vi "BBControl Dialog.vi"(8 "error in (no error)":errorcluster, 11 "BBCont Parameters In":T2 {"BBControl Criteria"."Comparison" items=["<", ">"]}) -> (0 "error out":errorcluster, 1 "Cancelled?":bool=TRUE, 2 "UI Refresh Needed?":bool, 3 "BBCont Parameters Out":T2 {"BBControl Criteria"."Comparison" items=["<", ">"]})   [LabVIEW 2024]
doc: "Dialog for selecting user specified settings."
uses:
  support/Control/BBControl Parameters.ctl
  ef7c00e2-4e74-40b8-8720-694a588d8cdf.vi
  74ebc26f-2795-41b4-bcda-487ba7bbdbc9.vi
  Display/Global 1.vi
  <vilib>/Utility/xml.llb/Write to XML File(string).vi
  <vilib>/Comparison/Equal/Equal Functor/Equal Functor.lvclass
panel:
  in  "Save as Preset":bool
  in  "Load Preset":bool
  in  "BangBang Control":T1(array[cluster]) {"Comparison" items=["<", ">"]}
  in  "Cancel Button":bool
  in  "OK Button":bool
  # "Non visible portion of dialog (needed for connector pane)."
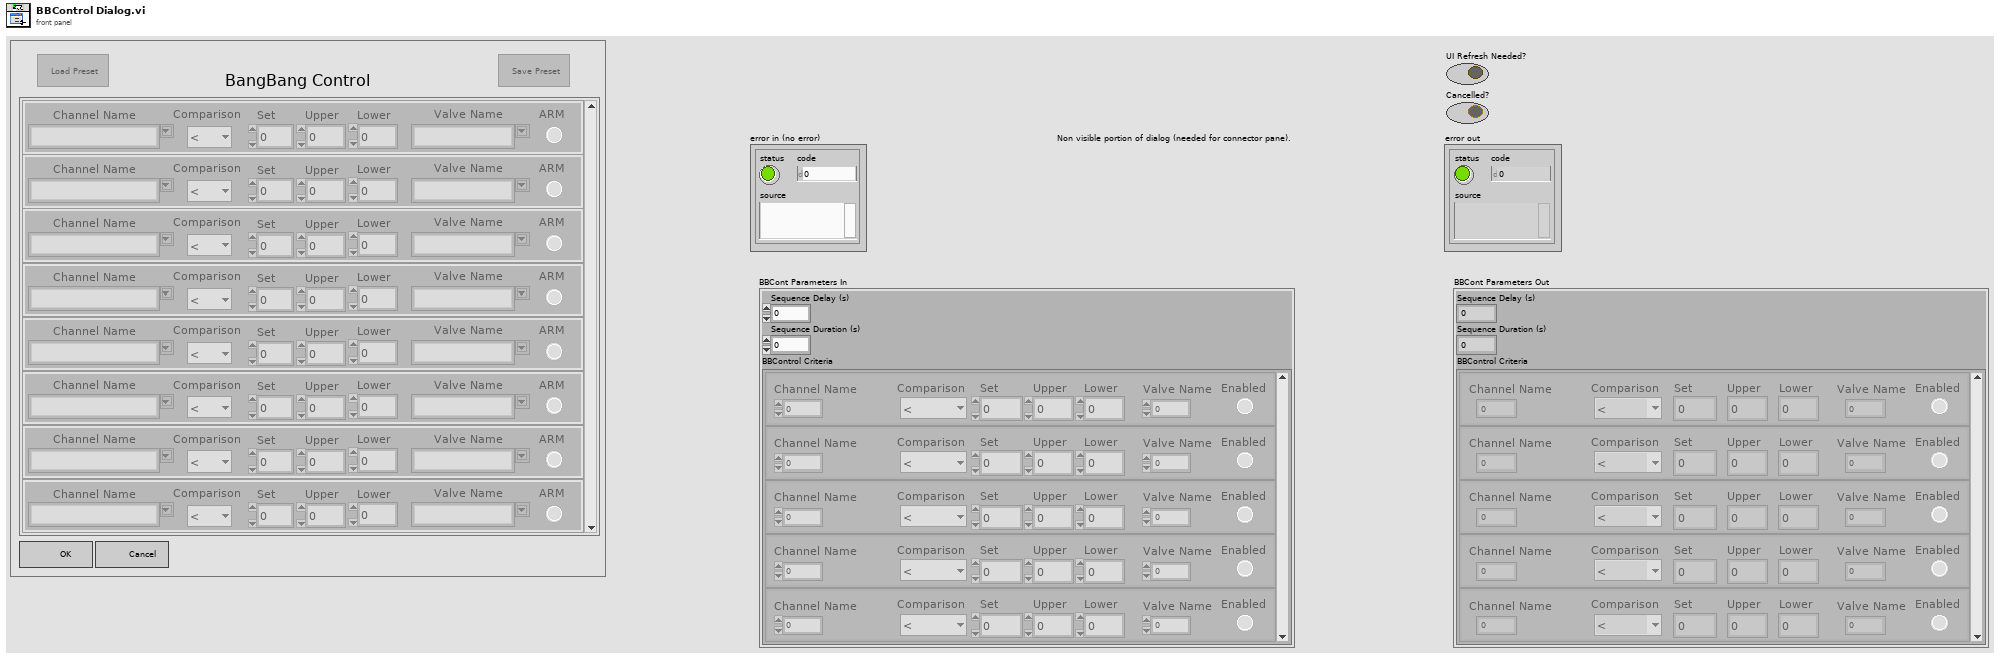
[diagram p1: front panel]
types:
  T1 = cluster{"Channel Name":string, "Comparison\n":u16, "Set":dbl, "ARM":bool, "Valve Name":string, "Upper":dbl, "Lower":dbl}[]
  T2 = typedef "BBControl Parameters.ctl" = cluster{"Sequence Delay (s)":dbl, "Sequence Duration (s)":dbl, "BBControl Criteria":cluster{"Channel Name":i32, "Comparison":u16, "Set":dbl, "Enabled":bool, "Valve Name":i32, "Upper":dbl, "Lower":dbl}[]}
  T3 = cluster{"Channel Name":string, "Comparison":u16, "Set":dbl, "Enabled":bool, "Valve Name":string, "Upper":dbl, "Lower":dbl}
  T4 = cluster{"Channel Name":i32, "Comparison":u16, "Set":dbl, "Enabled":bool, "Valve Name":i32, "Upper":dbl, "Lower":dbl}
  T5 = typedef "Calibration Configuration.ctl" = cluster{"ai Calibration Slope":dbl[], "ai Calibration Offset":dbl[], "ai Sensor Names ":string[], "tc Sensor Names":string[], "di Sensor Names":string[], "do Sensor Names":string[], "bc Sensor Names":string[], "ai Sensor Units":string[], "tc Sensor Units":string[], "bc Sensor Units":string[]}
  T6 = cluster{"Channel Name":i32, "Comparison":u16, "Set":dbl, "Enabled":bool, "Valve Name":i32, "Upper":dbl, "Lower":dbl}[]
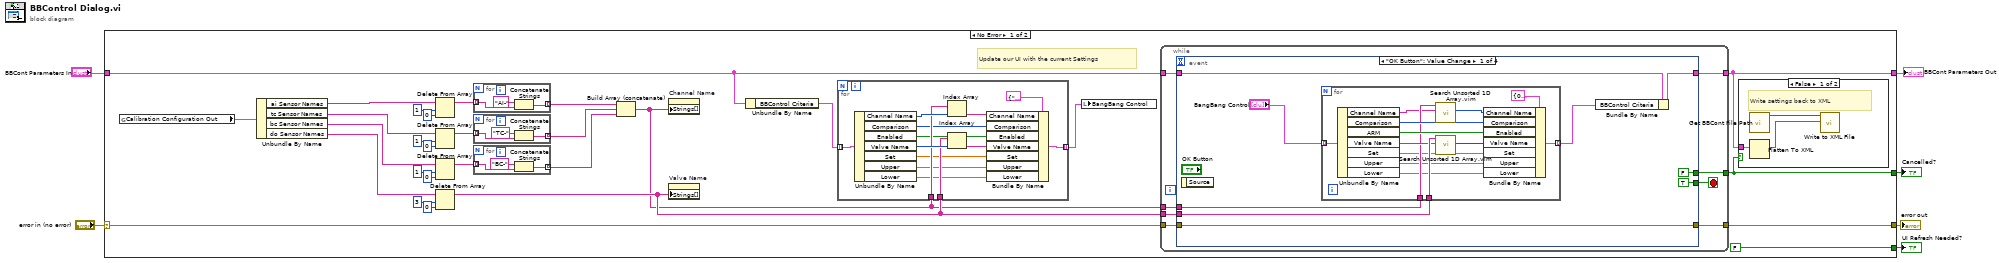
[diagram p0: block diagram]
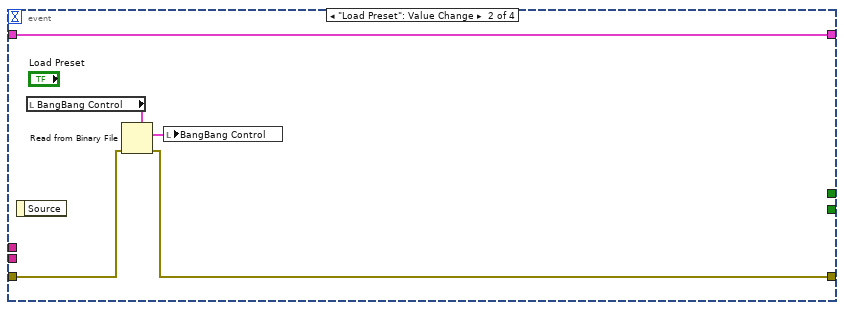
[diagram p3: hidden frame]
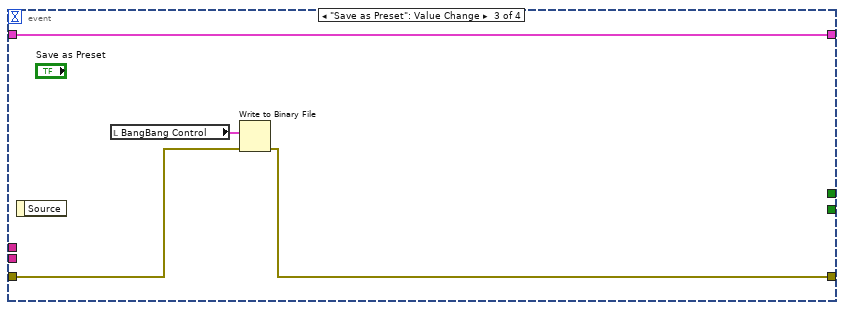
[diagram p4: hidden frame]
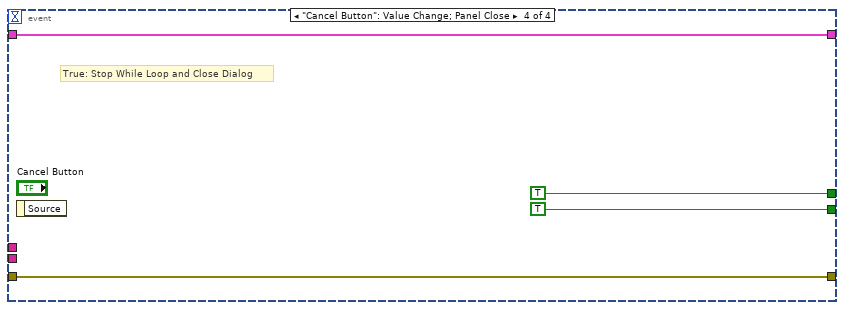
[diagram p5: hidden frame]
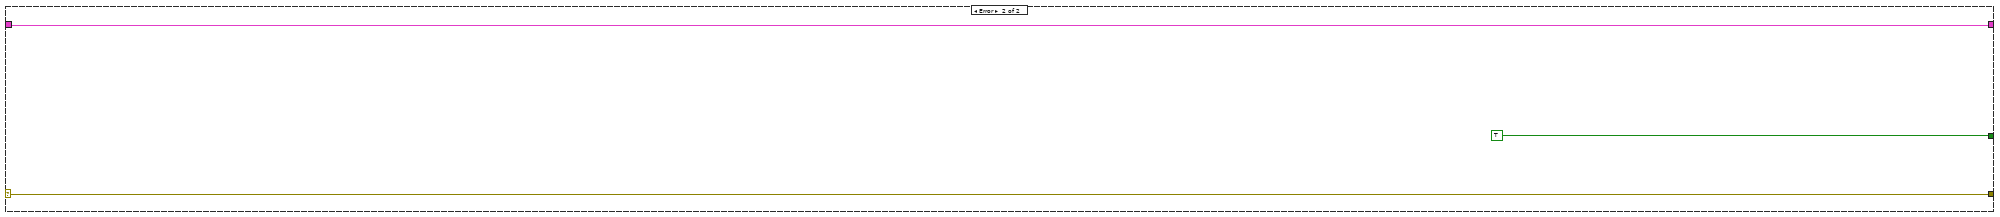
[diagram p6: hidden frame]
diagram:
  n1 = case shown="No Error" "error in (no error)" {
    selector: "error in (no error)" -> [w12 w108]
    tunnel: [w31 w108] -> w6
    tunnel: "BBCont Parameters In" -> [w34 w107]
    tunnel: [w33 w107] -> w1
    tunnel: [FALSE ("UI Refresh Needed?") _] -> w5
    tunnel: [w32 TRUE ("UI Refresh Needed?")] -> w4
    frame No Error {
      # "Update our UI with the current Settings"
      n2 = global read "Global 1.vi" "Calibration Configuration Out"() -> (w15:T5)
      n3 = Unbundle By Name(w15) -> ("ai Sensor Names"=w24:string[], "tc Sensor Names"=w23:string[], "bc Sensor Names"=w22:string[], "do Sensor Names"=w13:string[])
      n4 = Delete From Array(array=w24, length=1, index=0) -> (array with subset deleted=w19:string[])  [unwired: 1 out]
      n5 = Delete From Array(array=w23, length=1, index=0) -> (array with subset deleted=w20:string[])  [unwired: 1 out]
      n6 = Delete From Array(array=w22, length=1, index=0) -> (array with subset deleted=w21:string[])  [unwired: 1 out]
      n7 = Delete From Array(array=w13, length=3, index=0) -> (array with subset deleted=w9:string[])  [unwired: 1 out]
      n8 = for {
        tunnel: [w57] -> w18 mode=indexing
        tunnel: w19 -> [w56] mode=indexing
        n9 = Concatenate Strings("AI-" ("string"), w56) -> (w57:string)
      }
      n10 = for {
        tunnel: [w54] -> w17 mode=indexing
        tunnel: w20 -> [w53] mode=indexing
        n11 = Concatenate Strings("TC-" ("string"), w53) -> (w54:string)
      }
      n12 = for {
        tunnel: [w51] -> w16 mode=indexing
        tunnel: w21 -> [w50] mode=indexing
        n13 = Concatenate Strings("BC-" ("string"), w50) -> (w51:string)
      }
      n14 = Build Array (concatenate)(w18, w17, w16) -> (w8:string[])
      n15 = property on="Channel Name" class="CmbBox"("Strings[]"=w8) -> ()  [unwired: 2 in, 2 out]
      n16 = property on="Valve Name" class="CmbBox"("Strings[]"=w9) -> ()  [unwired: 2 in, 2 out]
      n17 = Unbundle By Name(w34) -> ("BBControl Criteria"=w11:T6)
      n18 = for {
        tunnel: w11 -> [w49] mode=indexing
        tunnel: [w48] -> w10 mode=indexing
        tunnel: w9 -> [w43]
        tunnel: w8 -> [w42]
        n19 = Unbundle By Name(w49) -> ("Channel Name"=w45:i32, "Comparison"=w40:u16, "Enabled"=w41:bool, "Valve Name"=w46:i32, "Set"=w38:dbl, "Upper"=w36:dbl, "Lower"=w37:dbl)
        n20 = Index Array(array=w42, index=w45) -> (element=w44:string)
        n21 = Index Array(array=w43, index=w46) -> (element=w47:string)
        n22 = Bundle By Name(cluster=T3 {"Channel Name"="", "Comparison"=0, "Set"=0.0, "Enabled"=FALSE, "Valve Name"="", "Upper"=0.0, "Lower"=0.0} ("Cluster"), "Channel Name"=w44, "Comparison"=w40, "Enabled"=w41, "Valve Name"=w47, "Set"=w38, "Upper"=w36, "Lower"=w37) -> (w48:T3)
      }
      n23 = local write "BangBang Control"(w10) -> ()
      n24 = while {
        tunnel: [w69] -> w32
        tunnel: [w68] -> w33
        tunnel: w34 -> [w67]
        tunnel: w12 -> [w65]
        tunnel: [w64] -> w31
        tunnel: w9 -> [w63]
        tunnel: w8 -> [w62]
        stop <- w66 stop-if-true
        n25 = event shown="[0] \"OK Button\": Value Change" {
          selector: _ -> [_ _ _ _]
          dyn-events: _ -> [_ _ _ _]
          timeout: _ -> [_ _ _ _]
          tunnel: [w75 w95 w101 w105] -> w68
          tunnel: w67 -> [w76 w95 w101 w105]
          tunnel: [FALSE ("UI Refresh Needed?") _ _ TRUE ("UI Refresh Needed?")] -> w69
          tunnel: [TRUE _ _ TRUE] -> w66
          tunnel: w65 -> [w74 w97 w100 w102]
          tunnel: [w74 w96 w99 w102] -> w64
          tunnel: w63 -> [w70 _ _ _]
          tunnel: w62 -> [w71 _ _ _]
          event "OK Button": Value Change {
            n26 = event-data() -> ()  [unwired: 1 in, 1 out]
            n27 = for {
              tunnel: "BangBang Control" -> [w92] mode=indexing
              tunnel: [w91] -> w72 mode=indexing
              tunnel: w70 -> [w86]
              tunnel: w71 -> [w84]
              n28 = Unbundle By Name(w92) -> ("Channel Name"=w83:string, "Comparison"=w87:u16, "ARM"=w88:bool, "Valve Name"=w85:string, "Set"=w81:dbl, "Upper"=w80:dbl, "Lower"=w79:dbl)
              n29 = call "Search Unsorted 1D Array.vim"("element"=w83, "unsorted 1D array"=w84) -> ("index of element"=w89:i32)  [unwired: 9 in]
              n30 = call "Search Unsorted 1D Array.vim"("element"=w85, "unsorted 1D array"=w86) -> ("index of element"=w90:i32)  [unwired: 9 in]
              n31 = Bundle By Name(cluster=T4 {"Channel Name"=0, "Comparison"=0, "Set"=0.0, "Enabled"=FALSE, "Valve Name"=0, "Upper"=0.0, "Lower"=0.0} ("Cluster"), "Channel Name"=w89, "Comparison"=w87, "Enabled"=w88, "Valve Name"=w90, "Set"=w81, "Upper"=w80, "Lower"=w79) -> (w91:T4)
            }
            n32 = Bundle By Name(cluster=w76, "BBControl Criteria"=w72) -> (w75:T2)
          }
          event "Load Preset": Value Change {
            n33 = event-data() -> ()  [unwired: 1 in, 1 out]
            n34 = local read "BangBang Control"() -> (w94:T1)
            n35 = Read from Binary File(5:w94, 8:w97) -> (0:w96:errorcluster, 2:w93:T1)  [unwired: 4 in, 2 out]
            n36 = local write "BangBang Control"(w93) -> ()
          }
          event "Save as Preset": Value Change {
            n37 = event-data() -> ()  [unwired: 1 in, 1 out]
            n38 = local read "BangBang Control"() -> (w98:T1)
            n39 = Write to Binary File(data=w98, error in=w100) -> (error out=w99:errorcluster)  [unwired: 4 in, 2 out]
          }
          event "Cancel Button": Value Change; Panel Close {
            # "True: Stop While Loop and Close Dialog"
            n40 = event-data() -> ()  [unwired: 1 in, 1 out]
          }
        }
      }
      n41 = case shown="False" w32 {
        tunnel: w33 -> [w61 _]
        frame False {
          # "Write settings back to XML"
          n42 = call "Get BBCont File Path.vi"() -> ("XML File Path"=w59:path)  [unwired: 10 in, 1 out]
          n43 = Flatten To XML(6:w61) -> (2:w60:string)
          n44 = call-poly <vilib>:"Write to XML File.vi"("XML Input"=w60, "XML File Path"=w59) -> ()  [unwired: 7 in, 3 out]
        }
        frame True {
        }
      }
    }
    frame Error {
    }
  }
  "UI Refresh Needed?" <- w5
  "error out" <- w6
  "Cancelled?" <- w4
  "BBCont Parameters Out" <- w1
